vi "AutoOneBallFront.vi"(8 "error in (no error)":errorcluster) -> (0 "error out":errorcluster)   [LabVIEW 2013]
uses:
  AutoStates.ctl
  AutoMode.ctl
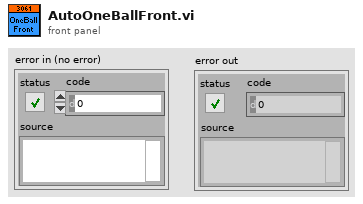
[diagram p1: front panel]
types:
  T1 = typedef "AutoStates.ctl" = enum16{"Init", "LowerArm", "CheckGoal", "Collect", "StopCollect", "RaiseServo", "Drive", "Wait", "ShootCollectorUp", "RaiseArm", "ShootCollectorDown", "Rotate1", "Rotate2", "Stop"}
  T2 = typedef "AutoMode.ctl" = enum16{"OneBallFront", "OneBallCollector", "TwoBallNormal", "TwoBallHot"}
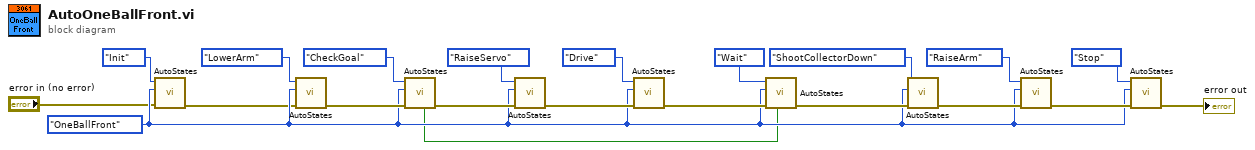
[diagram p0: block diagram]
diagram:
  w6 = AutoMode."OneBallFront" ("AutoMode")
  n1 = call "AutoStates.vi"("error in (no error)"="error in (no error)", "AutoMode"=w6, "AutoState"=AutoStates."Init") -> ("error out"=w1:errorcluster)  [unwired: 7 in, 1 out]
  n2 = call "AutoStates.vi"("error in (no error)"=w1, "AutoMode"=w6, "AutoState"=AutoStates."LowerArm") -> ("error out"=w18:errorcluster)  [unwired: 7 in, 1 out]
  n3 = call "AutoStates.vi"("error in (no error)"=w18, "AutoMode"=w6, "AutoState"=AutoStates."CheckGoal") -> ("error out"=w17:errorcluster, "Hot?"=w4:bool)  [unwired: 7 in]
  n4 = call "AutoStates.vi"("error in (no error)"=w17, "AutoMode"=w6, "AutoState"=AutoStates."RaiseServo") -> ("error out"=w9:errorcluster)  [unwired: 7 in, 1 out]
  n5 = call "AutoStates.vi"("error in (no error)"=w9, "AutoMode"=w6, "AutoState"=AutoStates."Drive") -> ("error out"=w7:errorcluster)  [unwired: 7 in, 1 out]
  n6 = call "AutoStates.vi"("WasHot?"=w4, "error in (no error)"=w7, "AutoMode"=w6, "AutoState"=AutoStates."Wait") -> ("error out"=w8:errorcluster)  [unwired: 6 in, 1 out]
  n7 = call "AutoStates.vi"("error in (no error)"=w8, "AutoMode"=w6, "AutoState"=AutoStates."ShootCollectorDown") -> ("error out"=w10:errorcluster)  [unwired: 7 in, 1 out]
  n8 = call "AutoStates.vi"("error in (no error)"=w10, "AutoMode"=w6, "AutoState"=AutoStates."RaiseArm") -> ("error out"=w12:errorcluster)  [unwired: 7 in, 1 out]
  n9 = call "AutoStates.vi"("error in (no error)"=w12, "AutoMode"=w6, "AutoState"=AutoStates."Stop") -> ("error out"=→"error out":errorcluster)  [unwired: 7 in, 1 out]
